vi "asset.update_commit.vi"(8 "error in":errorcluster, 11 "AssetUpdateStaging in":refnum<class "AssetUpdateStaging.lvclass">) -> (0 "error out":errorcluster, 3 "AssetUpdateStaging out":refnum<class "AssetUpdateStaging.lvclass">)   [LabVIEW 2020, in "AssetUpdateStaging.lvclass"]
doc: "Applies the staged changes to the asset with the given RID and returns a handle to the updated asset."
uses:
  AssetUpdateStaging.lvclass
  AssetUpdateStaging.lvclass/AssetUpdateStaging.ctl
  client.lvlib
panel:
  out "out_asset out":i32
  in  "rid":string
  in  "staging":i32
  in  "out_asset":i32
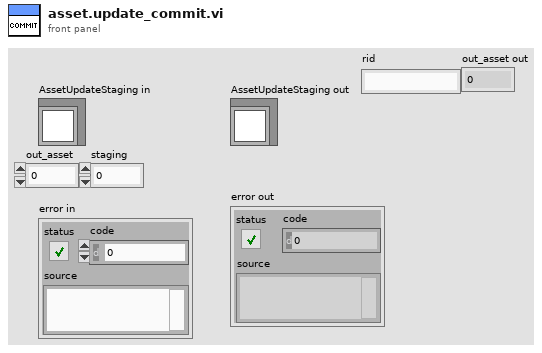
[diagram p1: front panel]
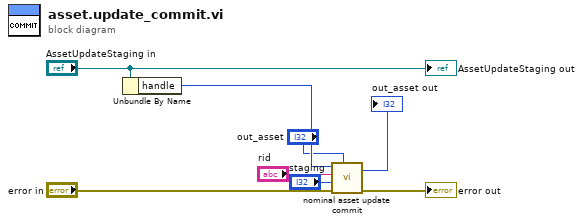
[diagram p0: block diagram]
diagram:
  n1 = Unbundle By Name("AssetUpdateStaging in") -> ("handle"=w6:i32)
  n2 = call "nominal asset update commit.vi"("out_asset"="out_asset", "error in (no error)"="error in", "staging"="staging", "rid"="rid", "client"=w6) -> ("error out"=→"error out":errorcluster, "out_asset out"=→"out_asset out":i32)  [unwired: 4 in, 1 out]
  "AssetUpdateStaging out" <- "AssetUpdateStaging in"
